vi "eSerial v000 - Kopya.vi"(2 "string to write":string="*IDN?", 3 "read":bool=TRUE, 4 "VISA resource name":refnum<visa-resource-name>="COM1") -> (0 "error out":errorcluster, 1 "read string":string)   [LabVIEW 2011]
doc: "The Advanced Serial Read and Write example performs a Serial Port Read, a Serial Port Write, or a combination of these actions while setting some advanced serial features like buffer size, termination characters, and XON/XOFF flow control. The user selects the actions (read or write) on the front panel. If both are selected, the VI will write the data first, read the data and then close the VISA session that is opened to the port. \n\nThe parameters set for the serial port must match the parameters of the connected instrument or device. In this example, the bytes to read parameter specifies the number of bytes that the serial port reads. If there were more bytes at the port than the number specified in bytes to read, those bytes would not be read. Also, if you specify to read more bytes than the number of bytes actually read, you might receive a timeout error message.\n\nINSTRUCTIONS:\n1) Select the serial resource and configuration parameters (baud rate, data bits, parity, stop bits, flow control).\n2) Termination character can be enabled and set. Also, set the required input buffer size prior to running the example.\n3) Select the operations to be performed. \n4) Connect the serial port to your device. If no device is available, perform a loopback test by doing one of the following. Short pins 2 and 3 on a RS-232 cable or short pin 4 to pin 8 and pin 5 to pin 9 on a RS-485/422 cable. \n5) Run the VI to see the data read. (The \"read string\" will match the \"string to write\" if a loopback test was performed.)\n\nThis example exposes several advanced features that you may need for your application. Not all applications need all the features shown in this example. The input buffer size is likely an important setting that you want to control in your application. This example expands upon the flow control option for XON and XOFF, allowing the user to choose those control characters. The timeout parameter has been brought to the front panel so a user can specify the time period the VISA Read will wait for the number of bytes to read before timing out. Also, the user has several controls for the termination character, which is discussed later.\n\nNote that you can press the write and read buttons and change the bytes to read parameters on the fly, while the example is running. However, you must stop the example to change the other configuration parameters after the example has started running, and then run again.\n\nSet the I/O buffer size slightly higher the amount of data you expect to receive. This is very important for applications that don't use flow control, as you may lose characters if the receive buffer overflows.\n\nSetting the timeout period ensures that the operation returns with a timeout error if the operation cannot be performed in the specified time period. \n\nSome devices require a termination character in order to identify the end of command strings. Some devices send a termination character to signify the end of data to be read. \n\nThis example shows how you can end the Read operation once a termination character is detected in the buffer and/or append a termination character at the end of the Write data. To enable the Read to end on a termination character, use the VISA Configure Serial Port or use the VISA Properties Serial End Mode for Reads, Termination Character Enable, and Termination Character. To end the Write with a termination character, use the VISA Properties Serial End Mode for Writes, the Send End Enable, and Termination Character. In this example, the same termination character is used for both the Read and the Write. You can specify two different characters for your application, if desired.\n\nYour application may require specific characters for the XON/XOFF Flow Control. You can specify these characters with the VISA Properties Flow Control XOFF Character and Flow Control XON Character. Note that if the standard XON and XOFF characters are used, then decimal 17 and 19 are unavailable for data values. Remember that using flow control and setting an adequate buffer size allow you to prevent buffer overflows."
uses:
  <vilib>/Instr/_visa.llb/VISA Set IO Buffer Mask.ctl
  <vilib>/Instr/_visa.llb/VISA Configure Serial Port (Instr).vi
panel:
  out "return count 2":u32
  out "return count":u32
  in  "write":bool=TRUE
  out "actual bytes read":u32
  # "On Windows/Linux, consider using the Instrument Driver Finder (Help>>Find Instrument Drivers) to search for an instrument driver for your instrument."
  # "Select the serial resource and the operations to be performed.  If all are selected, the VI will write the data first, read data and then close the VISA session that is opened to the port.  This VI will wait until the specified number of bytes is received at the port, until the timeout period is met, or until a termination character is received.  The default termination character in this example is the Line Feed ( ASCII 0xA, '\\n' ).  Also, set the required input buffer size prior to running the example.\nNote: The example loops until the STOP button is pressed."
  # "For additional information select File >> VI Properties >> Documentation"
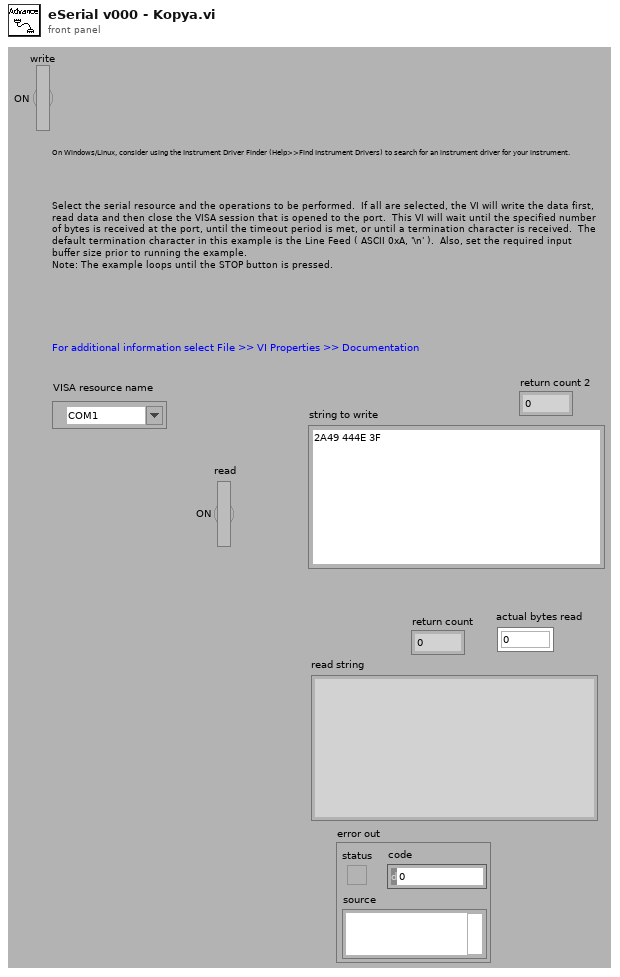
[diagram p1: front panel]
types:
  T1 = typedef "VISA Set IO Buffer Mask.ctl" = u16
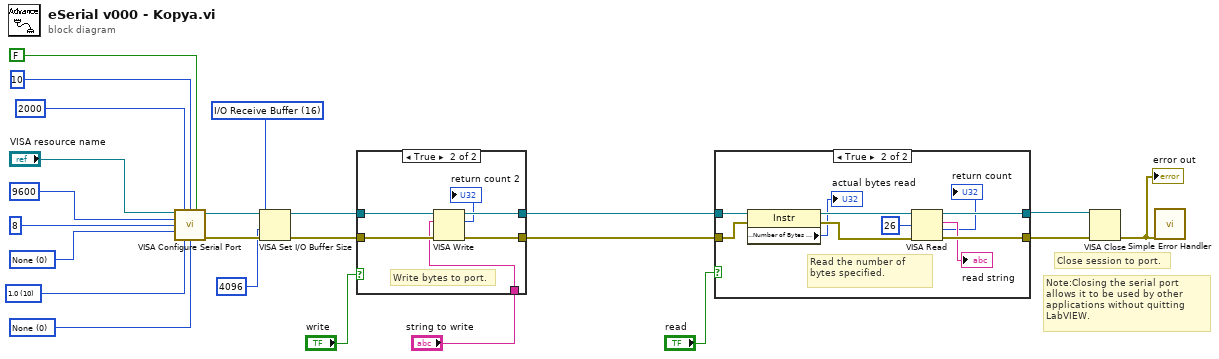
[diagram p0: block diagram]
diagram:
  w5 = T1 16 items=["I/O Receive Buffer"=16, "I/O Transmit Buffer"=32, "I/O Receive and Transmit Buffer"=48] ("Mask")
  w17 = u16 0 items=["None"=0, "XON/XOFF"=1, "RTS/CTS"=2, "DTR/DSR"=4] ("flow control")
  w20 = u16 10 items=["1.0"=10, "1.5"=15, "2.0"=20] ("stop bits")
  w21 = u16 0 items=["None", "Odd", "Even", "Mark", "Space"] ("parity")
  # "Note:Closing the serial port allows it to be used by other applications without quitting LabVIEW."
  # "Close session to port."
  n1 = call-poly "VISA Configure Serial Port"("VISA resource name"="VISA resource name", "timeout (10sec)"=u32 2000 ("timeout (ms)"), "termination char\n(0xA = '\\n' = LF)"=u8 10 ("termination char\n(0xA = '\\n' = LF)"), "Enable Termination\nChar (T)"=FALSE ("End read on termination character?"), "baud rate (9600)"=u32 9600 ("baud rate"), "data bits (8)"=u16 8 ("data bits"), "parity (0:none)"=w21, "stop bits (10: 1 bit)"=w20, "flow control (0:none)"=w17) -> ("VISA resource name out"=w9:refnum<visa-resource-name>, "error out"=w7:errorcluster)  [unwired: 1 in, 4 out]
  n2 = VISA Set I/O Buffer Size(VISA resource name=w9, mask (16)=w5, size (4096)=u32 4096, error in (no error)=w7) -> (VISA resource name out=w8:refnum<visa-resource-name>, error out=w6:errorcluster)
  n3 = case shown="True" "write" {
    tunnel: [w25 w31] -> w1
    tunnel: w8 -> [w24 w30]
    tunnel: w6 -> [w25 w29]
    tunnel: [w24 w28] -> w2
    tunnel: "string to write" -> [_ w27]
    frame False {
    }
    frame True {
      # "Write bytes to port."
      n4 = VISA Write(VISA resource name=w30, write buffer=w27, error in (no error)=w29) -> (VISA resource name out=w28:refnum<visa-resource-name>, return count=→"return count 2":u32, error out=w31:errorcluster)
    }
  }
  n5 = case shown="True" "read" {
    tunnel: w1 -> [w33 w39]
    tunnel: [w33 w43] -> w14
    tunnel: [w32 w42] -> w13
    tunnel: w2 -> [w32 w41]
    frame False {
    }
    frame True {
      # "Read the number of bytes specified."
      n6 = property class="Instr"(reference=w41, error in=w39) -> (reference out=w40:refnum<visa-resource-name>, error out=w38:errorcluster, "Serial Settings:Number of Bytes at Serial Port"=→"actual bytes read":u32)
      n7 = VISA Read(VISA resource name=w40, byte count=u32 26, error in (no error)=w38) -> (VISA resource name out=w42:refnum<visa-resource-name>, read buffer=→"read string":string, return count=→"return count":u32, error out=w43:errorcluster)
    }
  }
  n8 = VISA Close(VISA resource name=w13, error in (no error)=w14) -> (error out=w10:errorcluster)
  "error out" <- w10
  n9 = call <vilib>:"Simple Error Handler.vi"("error in (no error)"=w10) -> ()  [unwired: 1 in, 8 out]
